vi "RefNum Joystick.vi"() -> ()   [LabVIEW 2018]
panel:
  out "Joystick_1":string
  out "Joystick_0":string
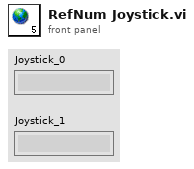
[diagram p1: front panel]
diagram:
